vi "cld 16 Jakub Wachowicz.vi"() -> ()   [LabVIEW 2018]
panel:
  in  "stop":bool
  in  "Control Panel Line Two":T1 {"Knob" scale=0.0..10.0}
  out "Display Value":T2
  out "Process Control":T3
  in  "Control Panel Line One":T1 {"Knob" scale=0.0..10.0}
  # "CLD 16"
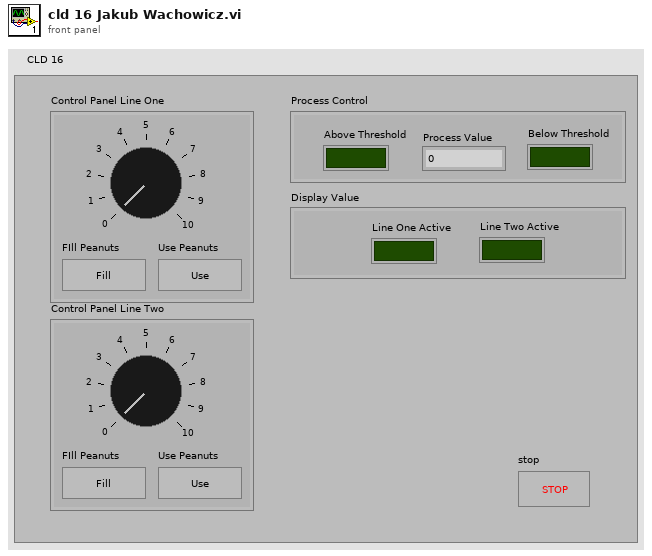
[diagram p1: front panel]
types:
  T1 = cluster{"Knob":dbl, "FIll Peanuts":bool, "Use Peanuts":bool}
  T2 = cluster{"Line One Active":bool, "Line Two Active":bool}
  T3 = cluster{"Above Threshold ":bool, "Below Threshold":bool, "Process Value":dbl}
  T4 = enum16{"Wait", "Fill CP 1", "Use CP1", "Fill CP 2", "Use CP 2"}
  T5 = enum16{"Wait", "Fill CP 1", "Use CP1", "Fill CP 2", "Use CP 2", "Stop", "Start"}
  T6 = enum8{"Enabled", "Disabled", "Disabled and Grayed Out"}
  T7 = enum16{"Wait", "Fill CP 1", "Use CP1", "Fill CP 2", "Use CP 2", "Stop"}
  T8 = cluster{dbl, "FIll Peanuts":bool, "Use Peanuts":bool}
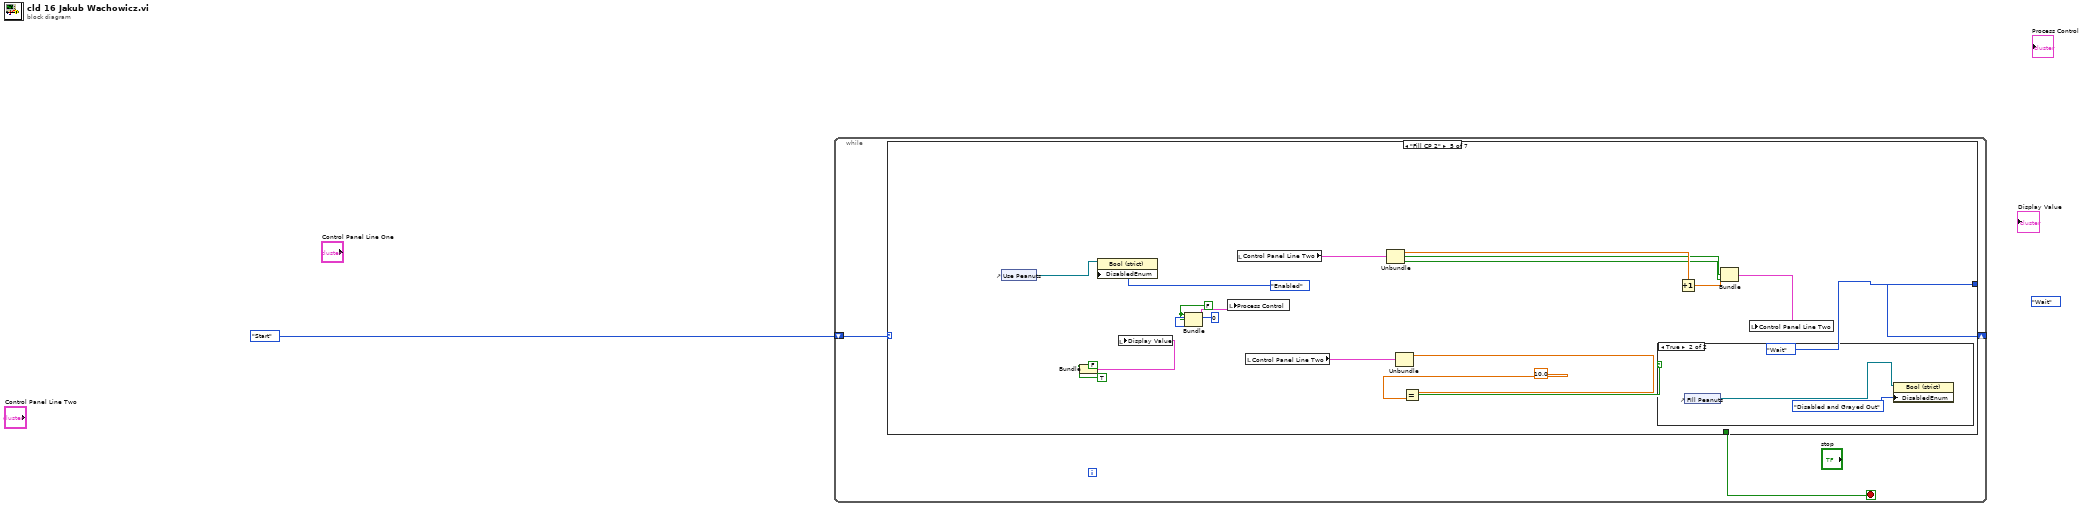
[diagram p0: block diagram]
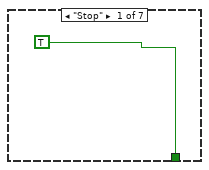
[diagram p2: hidden frame]
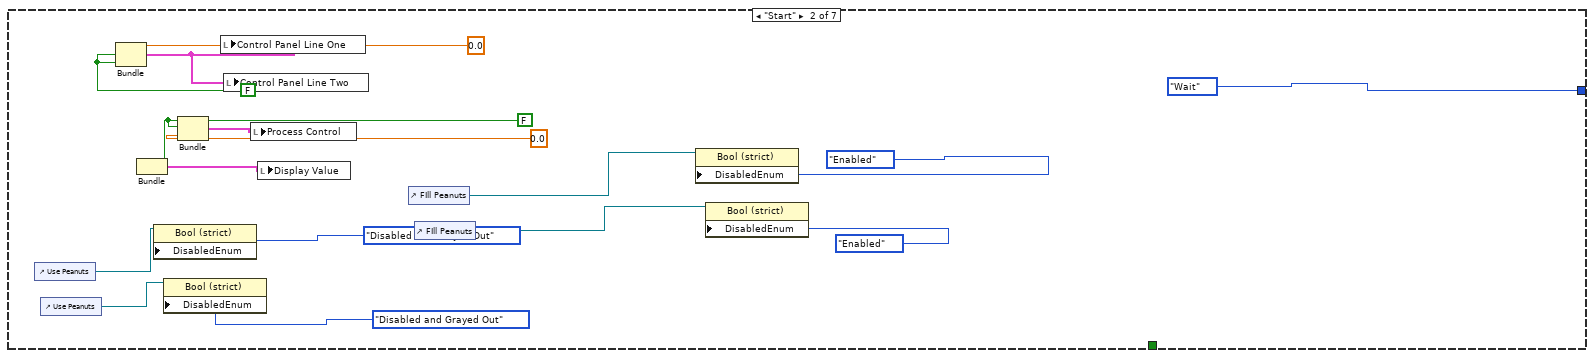
[diagram p3: hidden frame]
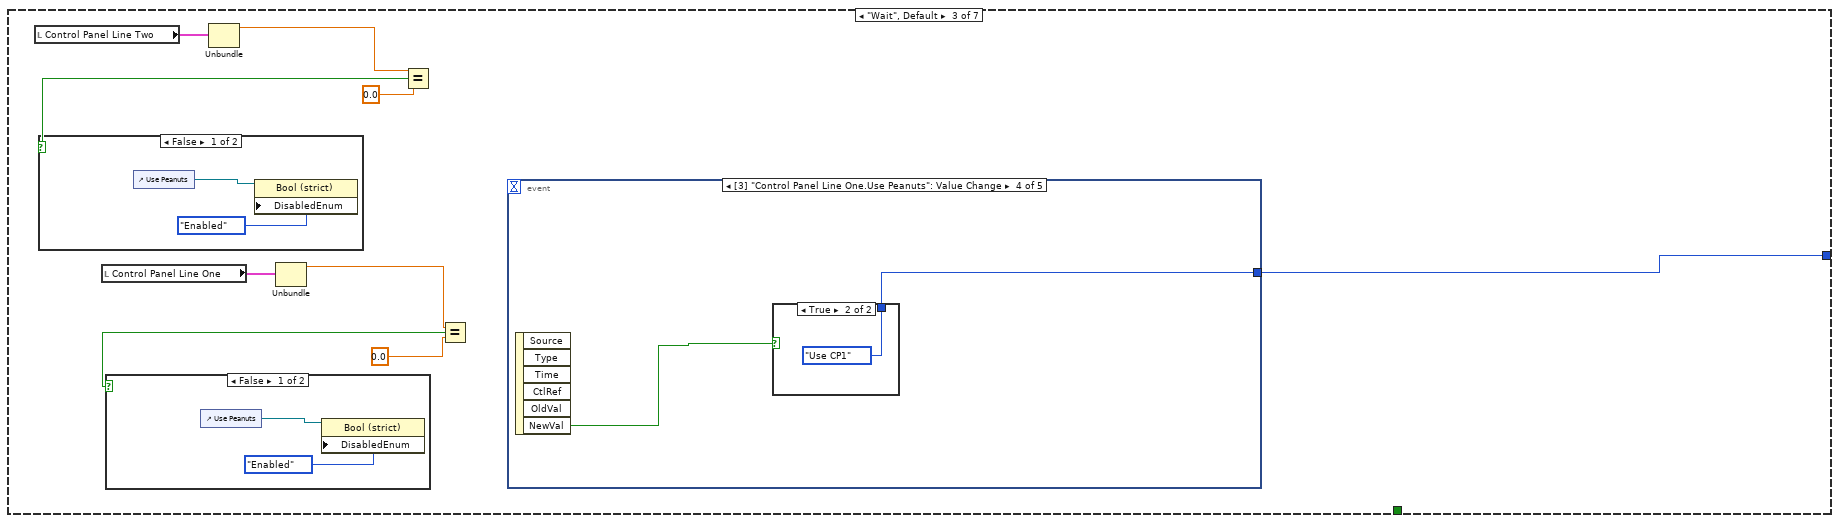
[diagram p4: hidden frame]
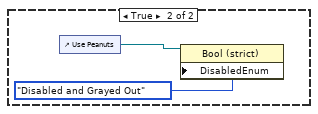
[diagram p5: hidden frame]
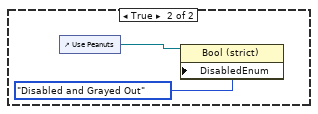
[diagram p6: hidden frame]
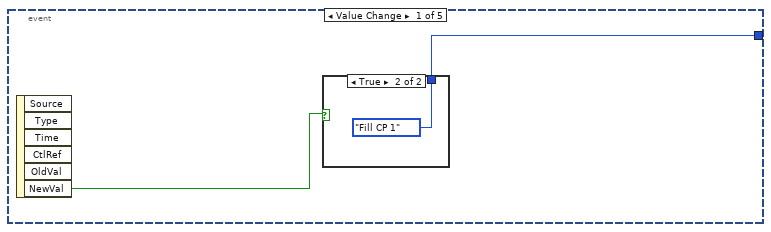
[diagram p7: hidden frame]
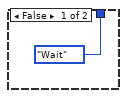
[diagram p8: hidden frame]
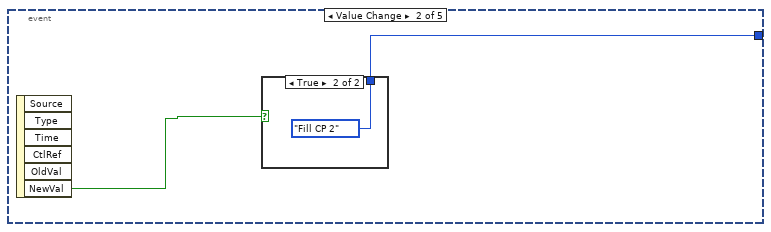
[diagram p9: hidden frame]
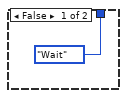
[diagram p10: hidden frame]
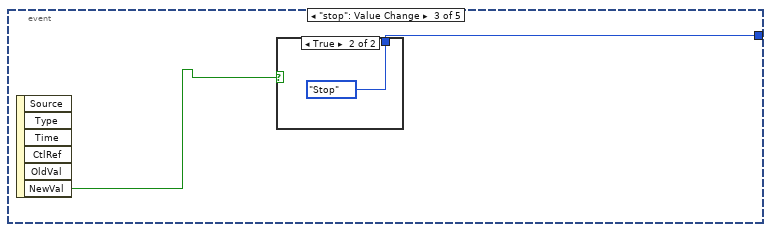
[diagram p11: hidden frame]
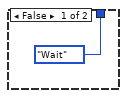
[diagram p12: hidden frame]
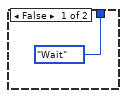
[diagram p13: hidden frame]
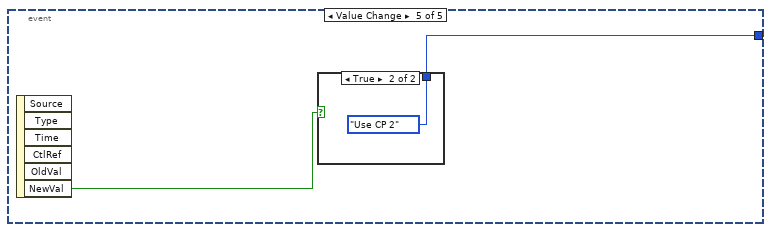
[diagram p14: hidden frame]
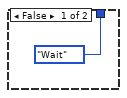
[diagram p15: hidden frame]
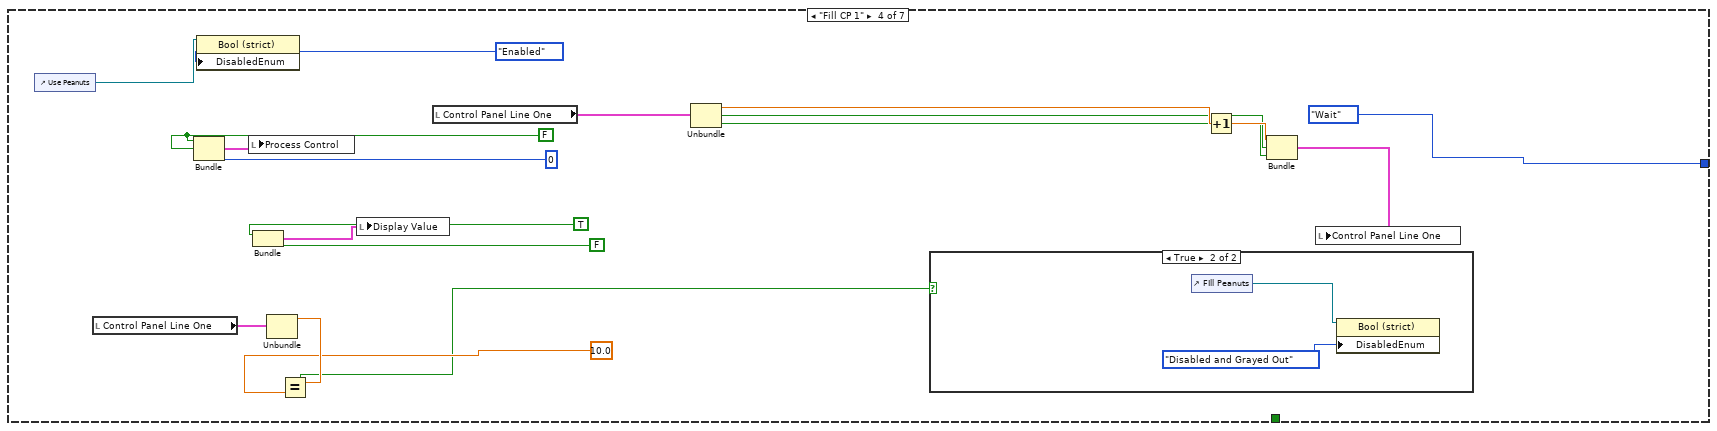
[diagram p16: hidden frame]
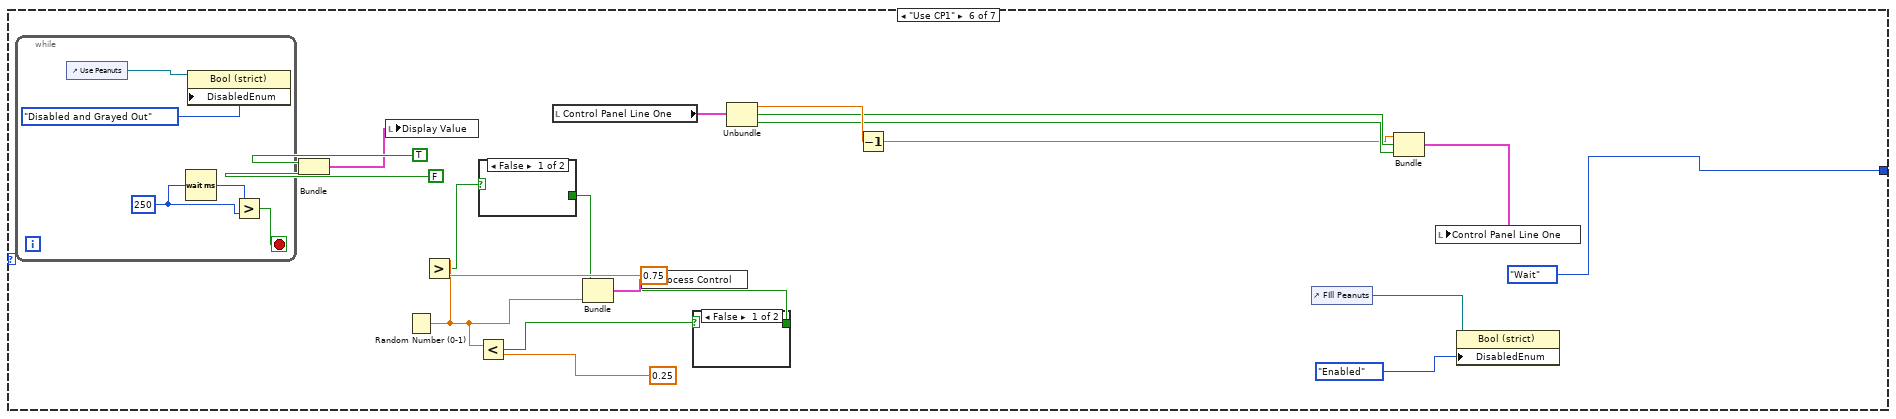
[diagram p19: hidden frame]
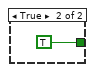
[diagram p20: hidden frame]
diagram:
  (unwired) T4."Wait"
  n1 = while {
    shift-right: [w4] -> _
    shift-left: T5."Start" -> [w3]
    stop <- w2 stop-if-true
    n2 = case shown="\"Fill CP 2\"" w3 {
      tunnel: [_ T5."Wait" w30 T4."Wait" T4."Wait" T4."Wait" T4."Wait"] -> w4
      tunnel: [TRUE _ _ _ _ _ _] -> w2
      frame "Stop" {
      }
      frame "Start" {
        w17 = FALSE
        w19 = FALSE
        n3 = control-ref of="Use Peanuts"() -> (w12:refnum<vi>)
        n4 = control-ref of="Use Peanuts"() -> (w13:refnum<vi>)
        n5 = Bundle(0.0, w19, w19) -> (w18:cluster{dbl, bool, bool})  [unwired: 1 in]
        n6 = Bundle(w17, w17) -> (w14:cluster{bool, bool})  [unwired: 1 in]
        n7 = property class="Bool (strict)"(reference=w12, "DisabledEnum"=T6."Disabled and Grayed Out" ("Disabled")) -> ()  [unwired: 1 in, 2 out]
        n8 = property class="Bool (strict)"(reference=w13, "DisabledEnum"=T6."Disabled and Grayed Out" ("Disabled")) -> ()  [unwired: 1 in, 2 out]
        n9 = Bundle(w17, w17, 0.0) -> (w15:cluster{bool, bool, dbl})  [unwired: 1 in]
        n10 = local write "Control Panel Line One"(w18) -> ()
        n11 = local write "Control Panel Line Two"(w18) -> ()
        n12 = local write "Process Control"(w15) -> ()
        n13 = local write "Display Value"(w14) -> ()
        n14 = control-ref of="FIll Peanuts"() -> (w9:refnum<vi>)
        n15 = control-ref of="FIll Peanuts"() -> (w8:refnum<vi>)
        n16 = property class="Bool (strict)"(reference=w9, "DisabledEnum"=T6."Enabled" ("Disabled")) -> ()  [unwired: 1 in, 2 out]
        n17 = property class="Bool (strict)"(reference=w8, "DisabledEnum"=T6."Enabled" ("Disabled")) -> ()  [unwired: 1 in, 2 out]
      }
      frame "Wait", Default {
        n18 = local read "Control Panel Line Two"() -> (w25:T1)
        n19 = local read "Control Panel Line One"() -> (w29:T1)
        n20 = Unbundle(w25) -> ("Knob"=w24:dbl)  [unwired: 2 out]
        n21 = Unbundle(w29) -> ("Knob"=w26:dbl)  [unwired: 2 out]
        n22 = Equal?(x=w24, y=0.0) -> (x = y?=w22:bool)
        n23 = case shown="False" w22 {
          frame False {
            n24 = control-ref of="Use Peanuts"() -> (w32:refnum<vi>)
            n25 = property class="Bool (strict)"(reference=w32, "DisabledEnum"=T6."Enabled" ("Disabled")) -> ()  [unwired: 1 in, 2 out]
          }
          frame True {
            n26 = control-ref of="Use Peanuts"() -> (w34:refnum<vi>)
            n27 = property class="Bool (strict)"(reference=w34, "DisabledEnum"=T6."Disabled and Grayed Out" ("Disabled")) -> ()  [unwired: 1 in, 2 out]
          }
        }
        n28 = Equal?(x=w26, y=0.0) -> (x = y?=w27:bool)
        n29 = case shown="False" w27 {
          frame False {
            n30 = control-ref of="Use Peanuts"() -> (w36:refnum<vi>)
            n31 = property class="Bool (strict)"(reference=w36, "DisabledEnum"=T6."Enabled" ("Disabled")) -> ()  [unwired: 1 in, 2 out]
          }
          frame True {
            n32 = control-ref of="Use Peanuts"() -> (w38:refnum<vi>)
            n33 = property class="Bool (strict)"(reference=w38, "DisabledEnum"=T6."Disabled and Grayed Out" ("Disabled")) -> ()  [unwired: 1 in, 2 out]
          }
        }
        n34 = event shown="[3] \"Control Panel Line One.Use Peanuts\": Value Change" {
          selector: _ -> [_ _ _ _ _]
          dyn-events: _ -> [_ _ _ _ _]
          timeout: _ -> [_ _ _ _ _]
          tunnel: [w39 w43 w47 w51 w55] -> w30
          event "Control Panel Line One.FIll Peanuts": Value Change {
            n35 = event-data() -> ("NewVal"=w40:bool)  [unwired: 1 in, 5 out]
            n36 = case shown="True" w40 {
              tunnel: [T4."Wait" T4."Fill CP 1"] -> w39
              frame False {
              }
              frame True {
              }
            }
          }
          event "Control Panel Line Two.FIll Peanuts": Value Change {
            n37 = event-data() -> ("NewVal"=w44:bool)  [unwired: 1 in, 5 out]
            n38 = case shown="True" w44 {
              tunnel: [T4."Wait" T4."Fill CP 2"] -> w43
              frame False {
              }
              frame True {
              }
            }
          }
          event "stop": Value Change {
            n39 = event-data() -> ("NewVal"=w48:bool)  [unwired: 1 in, 5 out]
            n40 = case shown="True" w48 {
              tunnel: [T4."Wait" T7."Stop"] -> w47
              frame False {
              }
              frame True {
              }
            }
          }
          event "Control Panel Line One.Use Peanuts": Value Change {
            n41 = event-data() -> ("NewVal"=w52:bool)  [unwired: 1 in, 5 out]
            n42 = case shown="True" w52 {
              tunnel: [T4."Wait" T4."Use CP1"] -> w51
              frame False {
              }
              frame True {
              }
            }
          }
          event "Control Panel Line Two.Use Peanuts": Value Change {
            n43 = event-data() -> ("NewVal"=w56:bool)  [unwired: 1 in, 5 out]
            n44 = case shown="True" w56 {
              tunnel: [T4."Wait" T4."Use CP 2"] -> w55
              frame False {
              }
              frame True {
              }
            }
          }
        }
      }
      frame "Fill CP 1" {
        w65 = FALSE
        n45 = control-ref of="Use Peanuts"() -> (w60:refnum<vi>)
        n46 = local read "Control Panel Line One"() -> (w63:T1)
        n47 = Bundle(w65, w65, 0) -> (w66:cluster{bool, bool, i32})  [unwired: 1 in]
        n48 = property class="Bool (strict)"(reference=w60, "DisabledEnum"=T6."Enabled" ("Disabled")) -> ()  [unwired: 1 in, 2 out]
        n49 = local write "Process Control"(w66) -> ()
        n50 = Bundle(TRUE, FALSE) -> (w68:cluster{bool, bool})  [unwired: 1 in]
        n51 = Unbundle(w63) -> ("Knob"=w64:dbl)  [unwired: 2 out]
        n52 = Equal?(x=w64, y=10.0) -> (x = y?=w61:bool)
        n53 = local write "Display Value"(w68) -> ()
        n54 = local read "Control Panel Line One"() -> (w77:T1)
        n55 = Unbundle(w77) -> ("Knob"=w76:dbl, "FIll Peanuts"=w74:bool, "Use Peanuts"=w73:bool)
        n56 = case shown="True" w61 {
          frame False {
          }
          frame True {
            n57 = control-ref of="FIll Peanuts"() -> (w78:refnum<vi>)
            n58 = property class="Bool (strict)"(reference=w78, "DisabledEnum"=T6."Disabled and Grayed Out" ("Disabled")) -> ()  [unwired: 1 in, 2 out]
          }
        }
        n59 = Increment(x=w76) -> (x+1=w75:dbl)
        n60 = Bundle(w75, "FIll Peanuts"=w74, "Use Peanuts"=w73) -> (w72:T8)  [unwired: 1 in]
        n61 = local write "Control Panel Line One"(w72) -> ()
      }
      frame "Fill CP 2" {
        w88 = FALSE
        n62 = control-ref of="Use Peanuts"() -> (w81:refnum<vi>)
        n63 = Bundle(FALSE, TRUE) -> (w90:cluster{bool, bool})  [unwired: 1 in]
        n64 = property class="Bool (strict)"(reference=w81, "DisabledEnum"=T6."Enabled" ("Disabled")) -> ()  [unwired: 1 in, 2 out]
        n65 = local write "Display Value"(w90) -> ()
        n66 = Bundle(w88, w88, 0) -> (w87:cluster{bool, bool, i32})  [unwired: 1 in]
        n67 = local write "Process Control"(w87) -> ()
        n68 = local read "Control Panel Line Two"() -> (w98:T1)
        n69 = local read "Control Panel Line Two"() -> (w84:T1)
        n70 = Unbundle(w98) -> ("Knob"=w97:dbl, "FIll Peanuts"=w96:bool, "Use Peanuts"=w95:bool)
        n71 = Unbundle(w84) -> ("Knob"=w85:dbl)  [unwired: 2 out]
        n72 = Equal?(x=w85, y=10.0) -> (x = y?=w82:bool)
        n73 = case shown="True" w82 {
          frame False {
          }
          frame True {
            n74 = control-ref of="FIll Peanuts"() -> (w99:refnum<vi>)
            n75 = property class="Bool (strict)"(reference=w99, "DisabledEnum"=T6."Disabled and Grayed Out" ("Disabled")) -> ()  [unwired: 1 in, 2 out]
          }
        }
        n76 = Increment(x=w97) -> (x+1=w86:dbl)
        n77 = Bundle(w86, "FIll Peanuts"=w96, "Use Peanuts"=w95) -> (w94:T8)  [unwired: 1 in]
        n78 = local write "Control Panel Line Two"(w94) -> ()
      }
      frame "Use CP1" {
        n79 = while {
          stop <- w122 stop-if-true
          w124 = u32 250 ("milliseconds to wait")
          n80 = control-ref of="Use Peanuts"() -> (w125:refnum<vi>)
          n81 = Wait (ms)(milliseconds to wait=w124) -> (millisecond timer value=w123:u32)
          n82 = property class="Bool (strict)"(reference=w125, "DisabledEnum"=T6."Disabled and Grayed Out" ("Disabled")) -> ()  [unwired: 1 in, 2 out]
          n83 = Greater?(x=w123, y=w124) -> (0:w122:bool)
        }
        n84 = Bundle(TRUE, FALSE) -> (w104:cluster{bool, bool})  [unwired: 1 in]
        n85 = local write "Display Value"(w104) -> ()
        n86 = Random Number (0-1)() -> (number: 0 to 1=w111:dbl)
        n87 = Greater?(x=w111, y=0.75) -> (0:w107:bool)
        n88 = Less?(x=w111, y=0.25) -> (x < y?=w110:bool)
        n89 = case shown="False" w107 {
          tunnel: [_ TRUE] -> w108
          frame False {
          }
          frame True {
          }
        }
        n90 = local read "Control Panel Line One"() -> (w120:T1)
        n91 = case shown="False" w110 {
          tunnel: [_ TRUE] -> w113
          frame False {
          }
          frame True {
          }
        }
        n92 = Bundle(w108, w113, "number: 0 to 1"=w111) -> (w114:cluster{bool, bool, "number: 0 to 1":dbl})  [unwired: 1 in]
        n93 = local write "Process Control"(w114) -> ()
        n94 = Unbundle(w120) -> ("Knob"=w119:dbl, "FIll Peanuts"=w118:bool, "Use Peanuts"=w117:bool)
        n95 = Decrement(x=w119) -> (x-1=w101:dbl)
        n96 = control-ref of="FIll Peanuts"() -> (w102:refnum<vi>)
        n97 = Bundle(w101, "FIll Peanuts"=w118, "Use Peanuts"=w117) -> (w116:T8)  [unwired: 1 in]
        n98 = local write "Control Panel Line One"(w116) -> ()
        n99 = property class="Bool (strict)"(reference=w102, "DisabledEnum"=T6."Enabled" ("Disabled")) -> ()  [unwired: 1 in, 2 out]
      }
      frame "Use CP 2" {
        n100 = while {
          stop <- w149 stop-if-true
          w151 = u32 250 ("milliseconds to wait")
          n101 = control-ref of="Use Peanuts"() -> (w152:refnum<vi>)
          n102 = Wait (ms)(milliseconds to wait=w151) -> (millisecond timer value=w150:u32)
          n103 = property class="Bool (strict)"(reference=w152, "DisabledEnum"=T6."Disabled and Grayed Out" ("Disabled")) -> ()  [unwired: 1 in, 2 out]
          n104 = Greater?(x=w150, y=w151) -> (0:w149:bool)
        }
        n105 = Random Number (0-1)() -> (number: 0 to 1=w138:dbl)
        n106 = Greater?(x=w138, y=0.75) -> (0:w134:bool)
        n107 = Less?(x=w138, y=0.25) -> (x < y?=w137:bool)
        n108 = case shown="True" w134 {
          tunnel: [_ TRUE] -> w135
          frame False {
          }
          frame True {
          }
        }
        n109 = Bundle(FALSE, TRUE) -> (w131:cluster{bool, bool})  [unwired: 1 in]
        n110 = local write "Display Value"(w131) -> ()
        n111 = case shown="True" w137 {
          tunnel: [_ TRUE] -> w140
          frame False {
          }
          frame True {
          }
        }
        n112 = Bundle(w135, w140, "number: 0 to 1"=w138) -> (w141:cluster{bool, bool, "number: 0 to 1":dbl})  [unwired: 1 in]
        n113 = local write "Process Control"(w141) -> ()
        n114 = local read "Control Panel Line Two"() -> (w147:T1)
        n115 = control-ref of="FIll Peanuts"() -> (w129:refnum<vi>)
        n116 = Unbundle(w147) -> ("Knob"=w146:dbl, "FIll Peanuts"=w145:bool, "Use Peanuts"=w144:bool)
        n117 = Decrement(x=w146) -> (x-1=w128:dbl)
        n118 = property class="Bool (strict)"(reference=w129, "DisabledEnum"=T6."Enabled" ("Disabled")) -> ()  [unwired: 1 in, 2 out]
        n119 = Bundle(w128, "FIll Peanuts"=w145, "Use Peanuts"=w144) -> (w143:T8)  [unwired: 1 in]
        n120 = local write "Control Panel Line Two"(w143) -> ()
      }
    }
  }
